vi "梦幻城堡C6~C20-Q6解析.vi"(11 "读取缓冲区":string) -> (3 "Status":T1)   [LabVIEW 2016, in "环境动力监测库.lvlib" / "UPS库.lvlib"]
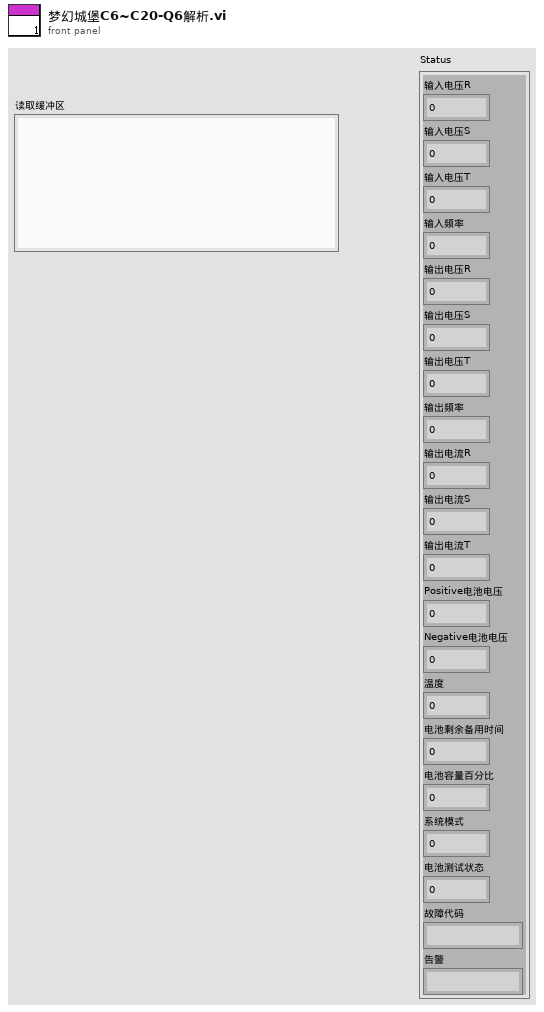
[diagram p1: front panel]
types:
  T1 = cluster{"输入电压R":dbl, "输入电压S":dbl, "输入电压T":dbl, "输入频率":dbl, "输出电压R":dbl, "输出电压S":dbl, "输出电压T":dbl, "输出频率":dbl, "输出电流R":dbl, "输出电流S":dbl, "输出电流T":dbl, "Positive电池电压":dbl, "Negative电池电压":dbl, "温度":dbl, "电池剩余备用时间":dbl, "电池容量百分比":dbl, "系统模式":dbl, "电池测试状态":dbl, "故障代码":string, "告警":string}
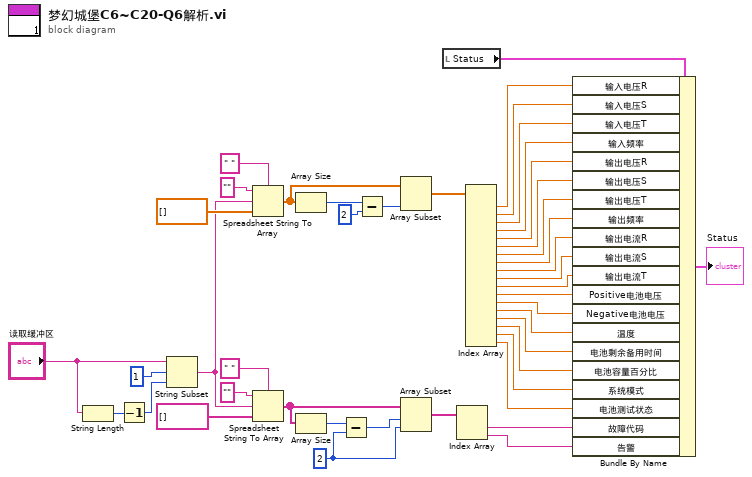
[diagram p0: block diagram]
diagram:
  w25 = 2 ("y")
  n1 = String Length(string="读取缓冲区") -> (length=w40:i32)
  n2 = Decrement(x=w40) -> (x-1=w39:i32)
  n3 = String Subset(string="读取缓冲区", offset (0)=1 ("偏移量(0)"), length (rest)=w39) -> (substring=w33:string)
  n4 = Spreadsheet String To Array(delimiter (Tab)=" " ("格式字符串"), format string="" ("格式字符串"), spreadsheet string=w33, array type (2D Dbl)=dbl[] []) -> (array=w32:dbl[])
  n5 = Spreadsheet String To Array(delimiter (Tab)=" " ("格式字符串"), format string="" ("格式字符串"), spreadsheet string=w33, array type (2D Dbl)=string[] []) -> (array=w27:string[])
  n6 = Array Size(array=w32) -> (size(s)=w31:i32)
  n7 = Array Size(array=w27) -> (size(s)=w28:i32)
  n8 = Subtract(x=w28, y=w25) -> (x-y=w26:i32)
  n9 = Subtract(x=w31, y=2) -> (x-y=w30:i32)
  n10 = Array Subset(array=w32, length=w30) -> (w23:dbl[])  [unwired: 1 in]
  n11 = Array Subset(array=w27, index=w26, length=w25) -> (w4:string[])
  n12 = local read "Status"() -> (w43:T1)
  n13 = Index Array(array=w4) -> (element #1=w3:string, element #2=w2:string)  [unwired: 2 in]
  n14 = Index Array(array=w23) -> (element #1=w22:dbl, element #2=w21:dbl, element #3=w20:dbl, element #4=w19:dbl, element #5=w18:dbl, element #6=w17:dbl, element #7=w16:dbl, element #8=w15:dbl, element #9=w14:dbl, element #10=w13:dbl, element #11=w12:dbl, element #12=w11:dbl, element #13=w10:dbl, element #14=w9:dbl, element #15=w8:dbl, element #16=w7:dbl, element #17=w6:dbl, element #18=w5:dbl)  [unwired: 18 in]
  n15 = Bundle By Name(cluster=w43, "输入电压R"=w22, "输入电压S"=w21, "输入电压T"=w20, "输入频率"=w19, "输出电压R"=w18, "输出电压S"=w17, "输出电压T"=w16, "输出频率"=w15, "输出电流R"=w14, "输出电流S"=w13, "输出电流T"=w12, "Positive电池电压"=w11, "Negative电池电压"=w10, "温度"=w9, "电池剩余备用时间"=w8, "电池容量百分比"=w7, "系统模式"=w6, "电池测试状态"=w5, "故障代码"=w3, "告警"=w2) -> (→"Status":T1)
